vi "Write cmd to skywire serial.vi"(8 "error in (no error)":errorcluster, 9 "Wait after write (1000 msecs)":u32=1000, 10 "write buffer":string, 11 "VISA Refnum in":refnum<visa-resource-name>) -> (0 "error out":errorcluster, 3 "VISA Refnum out":refnum<visa-resource-name>)   [LabVIEW 2013]
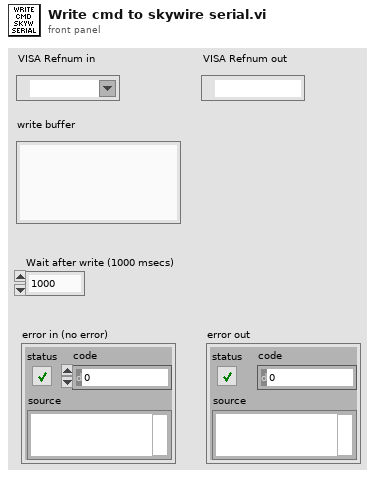
[diagram p1: front panel]
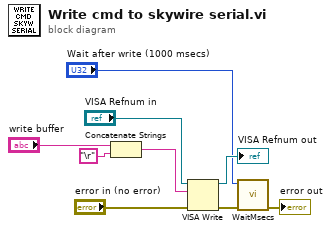
[diagram p0: block diagram]
diagram:
  n1 = Concatenate Strings("write buffer", "\r") -> (w4:string)
  n2 = VISA Write(VISA resource name="VISA Refnum in", write buffer=w4, error in (no error)="error in (no error)") -> (VISA resource name out=→"VISA Refnum out":refnum<visa-resource-name>, error out=w3:errorcluster)  [unwired: 1 out]
  n3 = call "WaitMsecs.vi"("error in (no error)"=w3, "Wait Msecs"="Wait after write (1000 msecs)") -> ("error out"=→"error out":errorcluster)  [unwired: 9 in]
